vi "Bye Bye.vi"(8 "Objects":T1[](array[typedef]) {"Aspect Ratio" format="%.2f"}) -> (0 "Count":i16)   [LabVIEW 2015]
uses:
  TypeDefs Host/Object Info.ctl
  TypeDefs Host/Counter FGV Enum.ctl
  TypeDefs Host/Timer Enum.ctl
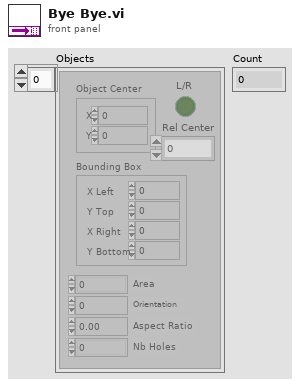
[diagram p1: front panel]
types:
  T1 = typedef "Object Info.ctl" = cluster{"Object Center":cluster{"X":u16, "Y":u16}, "Bounding Box":cluster{"X Left":u16, "Y Top":u16, "X Right":u16, "Y Bottom":u16}, "Area":u16, "Orientation":u16, "Aspect Ratio":sgl, "Nb Holes":u16, "L/R":bool, "Rel Center":u16}
  T2 = typedef "Counter FGV Enum.ctl" = enum16{"Get Count", "Set Count"}
  T3 = typedef "Timer Enum.ctl" = enum16{"Timestamp", "Get Period", "Last Period"}
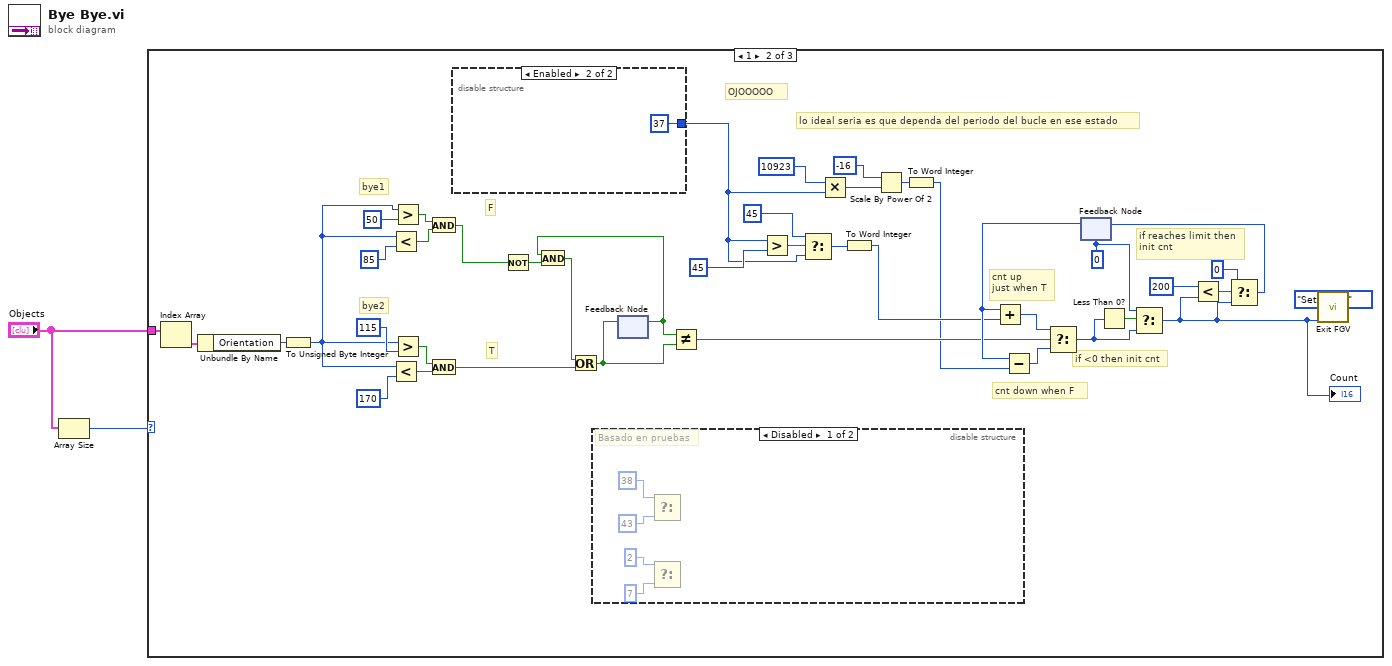
[diagram p0: block diagram]
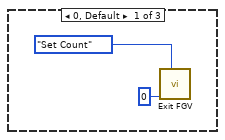
[diagram p2: hidden frame]
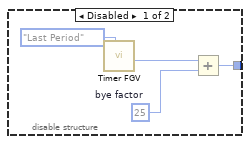
[diagram p3: hidden frame]
diagram:
  n1 = Array Size(array="Objects") -> (size(s)=w1:i32)
  n2 = case shown="1" w1 {
    tunnel: "Objects" -> [_ w19 _]
    frame 0, Default {
      n3 = call "Exit FGV.vi"("Exit FGV Command"=Counter_FGV_Enum."Set Count", "Count In"=i16 0) -> ()  [unwired: 9 in, 1 out]
    }
    frame 1 {
      w26 = i16 0
      # "OJOOOOO"
      # "if reaches limit then\ninit cnt"
      # "if <0 then init cnt"
      # "cnt down when F"
      # "cnt up\njust when T"
      # "lo ideal seria es que dependa del periodo del bucle en ese estado"
      # "bye2"
      # "bye1"
      # "T"
      # "F"
      n4 = Index Array(array=w19) -> (element=w18:T1)  [unwired: 1 in]
      n5 = Unbundle By Name(w18) -> ("Orientation"=w17:u16)
      n6 = To Unsigned Byte Integer(number=w17) -> (unsigned 8bit integer=w29:u8)
      n7 = Less?(x=w29, y=u8 85) -> (x < y?=w38:bool)
      n8 = Less?(x=w29, y=u8 170) -> (x < y?=w44:bool)
      n9 = Greater?(x=w29, y=u8 50) -> (0:w37:bool)
      n10 = Greater?(x=w29, y=u8 115) -> (0:w43:bool)
      n11 = And(x=w37, y=w38) -> (x .and. y?=w39:bool)
      n12 = And(x=w43, y=w44) -> (x .and. y?=w46:bool)
      n13 = disable-structure shown="Enabled" {
        disable-tunnel: [w48 u32 37] -> w5
        frame Disabled {
          w47 = u32 25  # bye factor
          n14 = call "Timer FGV.vi"("Timer Command"=Timer_Enum."Last Period") -> ("Period"=w50:u32)  [unwired: 9 in, 1 out]
          n15 = Add(x=w50, y=w47) -> (x+y=w48:u32)
        }
        frame Enabled {
        }
      }
      n16 = Not(x=w39) -> (.not. x?=w40:bool)
      n17 = disable-structure shown="Disabled" {
        frame Disabled {
          # "Basado en pruebas"
          n18 = Select(t=i16 38, f=i16 43) -> ()  [unwired: 1 in, 1 out]
          n19 = Select(t=i16 2, f=i16 7) -> ()  [unwired: 1 in, 1 out]
        }
        frame Enabled {
        }
      }
      n20 = feedback #1() -> (w30:bool)  [unwired: 1 in]
      n21 = And(x=w30, y=w40) -> (x .and. y?=w41:bool)
      n22 = Or(x=w41, y=w46) -> (x .or. y?=w42:bool)
      n23 = feedback-in #1(w42) -> ()
      n24 = Not Equal?(x=w30, y=w42) -> (x != y?=w27:bool)
      n25 = Greater?(x=w5, y=u32 45) -> (0:w11:bool)
      n26 = Select(t=u32 45, s=w11, f=w5) -> (s? t:f=w13:u32)
      n27 = Multiply(x=u32 10923, y=w5) -> (x*y=w14:u32)
      n28 = To Word Integer(number=w13) -> (16bit integer=w8:i16)
      n29 = Scale By Power Of 2(n=i16 -16, x=w14) -> (x*2^n=w10:u32)
      n30 = To Word Integer(number=w10) -> (16bit integer=w7:i16)
      n31 = feedback #2(w26) -> (w34:i16)
      n32 = Add(x=w34, y=w8) -> (x+y=w32:i16)
      n33 = Subtract(x=w34, y=w7) -> (x-y=w35:i16)
      n34 = Select(t=w32, s=w27, f=w35) -> (s? t:f=w24:i16)
      n35 = Less Than 0?(x=w24) -> (x < 0?=w25:bool)
      n36 = Select(t=w26, s=w25, f=w24) -> (s? t:f=w6:i16)
      "Count" <- w6
      n37 = Less?(x=i16 200, y=w6) -> (x < y?=w23:bool)
      n38 = Select(t=i16 0, s=w23, f=w6) -> (s? t:f=w21:i16)
      n39 = feedback-in #2(w21) -> ()
      n40 = call "Exit FGV.vi"("Exit FGV Command"=Counter_FGV_Enum."Set Count", "Count In"=w6) -> ()  [unwired: 9 in, 1 out]
    }
    frame 2 {
      # "Other Gestures"
    }
  }
